vi "libdaq_adc_set_sample_parameter.vi"(0 "error in (no error)":errorcluster, 1 "device_name":string, 2 "module_name":string, 4 "adc_samplepara":T1={"channel_list "=[1], "channel_count"=0, "sample_mode"=0, "frequency"=0, "cycles"=1, "group_interval"=1}) -> (14 "error out":errorcluster, 15 "device_name":string, 16 "module_name":string)   [LabVIEW 2022 SP3, in "libdaqVI.lvlib"]
doc: "配置ADC模块的采样模式和参数，包括采样通道、采样频率和采样模式采等，采样参数由samplepara指向的结构中指定"
uses:
  libdaqVI.lvlib
  dll/daqlib.dll
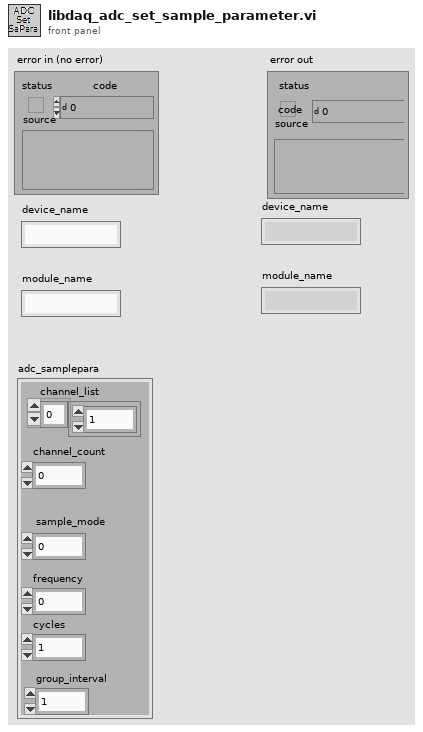
[diagram p1: front panel]
types:
  T1 = cluster{"channel_list ":u8[], "channel_count":u8, "sample_mode":u8, "frequency":u32, "cycles":u32, "group_interval":u32}
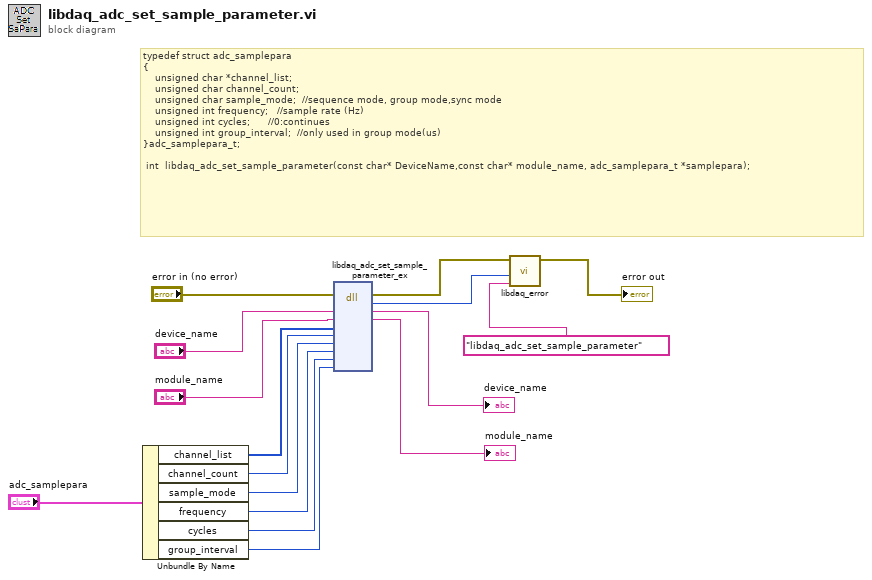
[diagram p0: block diagram]
diagram:
  # "typedef struct adc_samplepara\n{\n    unsigned char *channel_list;\n    unsigned char channel_count;\n    unsigned char sample_mode;  //sequence mode, group mode,sync mode\n    unsigned int frequency;   //sample rate (Hz)\n    unsigned int cycles;      //0:continues\n    unsigned int group_interval;  //only used in group mode(us)\n}adc_samplepara_t;\n\n int  libdaq_adc_set_sample_parameter(const char* DeviceName,const char* module_name, adc_samplepara_t *samplepara);"
  n1 = Unbundle By Name("adc_samplepara") -> ("channel_list"=w10:u8[], "channel_count"=w9:u8, "sample_mode"=w8:u8, "frequency"=w7:u32, "cycles"=w6:u32, "group_interval"=w5:u32)
  n2 = dll-call lib="D:/Labview_projects/DAQ_USB3212/libdaqVI/dll/daqlib.dll" fn="libdaq_adc_set_sample_parameter_ex"(error in="error in (no error)", "device_name"="device_name", "module_name"="module_name", "channel_list"=w10, "channel_count"=w9, "sample_mode"=w8, "frequency"=w7, "cycles"=w6, "group_interval"=w5) -> (error out=w4:errorcluster, "return type"=w2:i32, "device_name"=→"device_name":string, "module_name"=→"module_name":string)  [unwired: 8 in, 1 out]
  n3 = call "libdaq_error.vi"("error source"="libdaq_adc_set_sample_parameter", "error code"=w2, "错误输入（无错误）"=w4) -> ("错误输出"=→"error out":errorcluster)  [unwired: 8 in]
